vi "Generate Non Text Layer(s).vi"(0 "Library Path":path, 5 "new picture":picture, 7 "VI Refnum in":refnum<vi>, 11 "error in":errorcluster) -> (4 "Layers":refnum<class "Layer.lvclass">[](array[class]), 6 "Icon Height":i16, 15 "error out":errorcluster)   [LabVIEW 2024, in "Text-Based VI Icon.lvlib"]
uses:
  <vilib>/LabVIEW Icon API/Set Text Icon/Text-Based VI Icon.lvlib
  <vilib>/LabVIEW Icon API/lv_icon/Classes/Layer/Layer.lvclass
  <vilib>/LabVIEW Icon API/lv_icon/Controls/Layer.ctl
  <vilib>/LabVIEW Icon API/Set Text Icon/User Visible Strings.vi
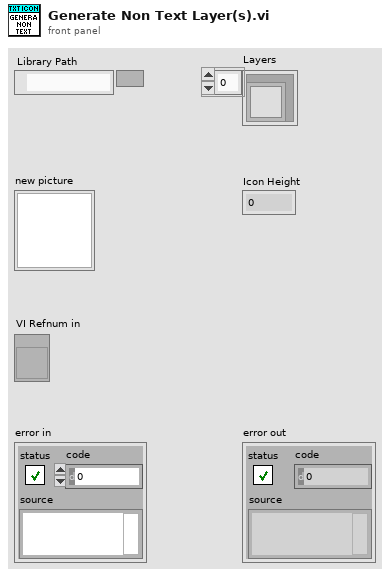
[diagram p1: front panel]
types:
  T1 = cluster{"left":i16, "top":i16, "right":i16, "bottom":i16}
  T2 = typedef "Layer.ctl" = cluster{"LayerIcon":picture, "LayerName":string, "Opacity":u8, "Visibility?":bool}
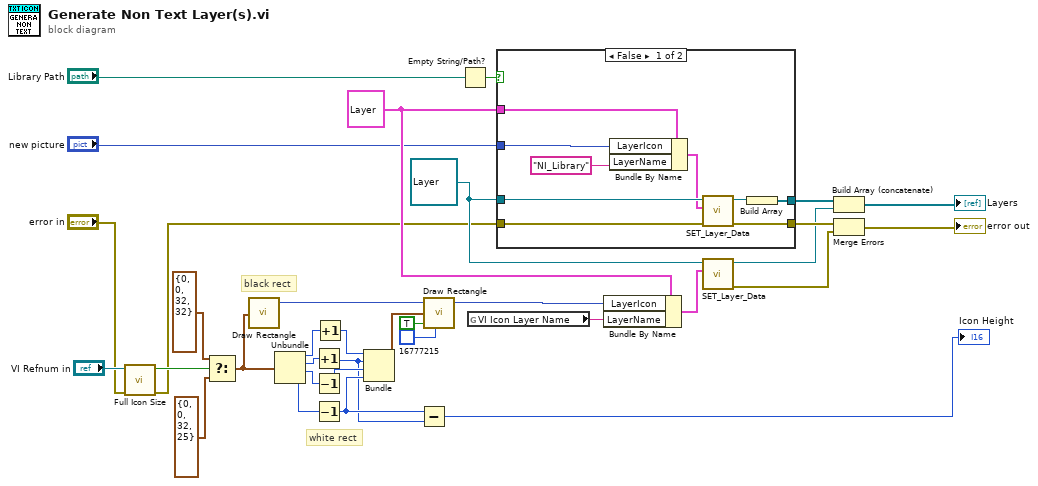
[diagram p0: block diagram]
diagram:
  w22 = T2 {"LayerIcon"=bytes[3102], "LayerName"="", "Opacity"=100, "Visibility?"=TRUE} ("Data")
  w33 = refnum<class "Layer.lvclass"> refnum ("Layer.lvclass in")
  # "black rect"
  # "white rect"
  n1 = call <vilib>:"Full Icon Size.vi"("error in"="error in", "VI in"="VI Refnum in") -> ("error out"=w1:errorcluster, "Full Icon Size?"=w12:bool)  [unwired: 8 in]
  n2 = Select(t=T1 {"left"=0, "top"=0, "right"=32, "bottom"=32} ("rect"), s=w12, f=T1 {"left"=0, "top"=0, "right"=32, "bottom"=25} ("rect")) -> (s? t:f=w21:T1)
  n3 = call <vilib>:"Draw Rectangle.vi"("rect"=w21) -> ("new picture"=w32:picture)  [unwired: 8 in]
  n4 = Unbundle(w21) -> ("left"=w20:i16, "top"=w19:i16, "right"=w18:i16, "bottom"=w11:i16)
  n5 = Increment(x=w19) -> (x+1=w9:i16)
  n6 = Decrement(x=w18) -> (x-1=w16:i16)
  n7 = Decrement(x=w11) -> (x-1=w10:i16)
  n8 = Increment(x=w20) -> (x+1=w17:i16)
  n9 = Bundle(w17, w9, w16, w10) -> (w15:cluster{i16, i16, i16, i16})  [unwired: 1 in]
  n10 = Subtract(x=w10, y=w9) -> (x-y=→"Icon Height":i16)
  n11 = call <vilib>:"Draw Rectangle.vi"("picture"=w32, "rect"=w15, "fill?(F)"=TRUE, "color(black)"=u32 16777215) -> ("new picture"=w31:picture)  [unwired: 5 in]
  n12 = Empty String/Path?(string/path="Library Path") -> (empty?=w34:bool)
  n13 = global read "User Visible Strings.vi" "VI Icon Layer Name"() -> (w27:string)
  n14 = case shown="False" w34 {
    tunnel: w1 -> [w41 w44]
    tunnel: w33 -> [w43 _]
    tunnel: w22 -> [w42 _]
    tunnel: [w37 w44] -> w26
    tunnel: [w36 _] -> w24
    tunnel: "new picture" -> [w35 _]
    frame False {
      n15 = Bundle By Name(cluster=w42, "LayerIcon"=w35, "LayerName"="NI_Library") -> (w40:T2)
      n16 = call-dynamic "SET_Layer_Data.vi"("error in (no error)"=w41, "Data"=w40, "Layer.lvclass in"=w43) -> ("error out"=w37:errorcluster, "Layer.lvclass out"=w38:refnum<class "Layer.lvclass">)  [unwired: 7 in]
      n17 = Build Array(w38) -> (w36:refnum<class "Layer.lvclass">[])
    }
    frame True {
    }
  }
  n18 = Bundle By Name(cluster=w22, "LayerIcon"=w31, "LayerName"=w27) -> (w28:T2)
  n19 = call-dynamic "SET_Layer_Data.vi"("Data"=w28, "Layer.lvclass in"=w33) -> ("error out"=w25:errorcluster, "Layer.lvclass out"=w23:refnum<class "Layer.lvclass">)  [unwired: 8 in]
  n20 = Build Array (concatenate)(w24, w23) -> (→"Layers":refnum<class "Layer.lvclass">[])
  n21 = Merge Errors(w26, w25) -> (→"error out":errorcluster)
